vi "1_Search string and replace.vi"() -> ()   [LabVIEW 2010]
panel:
  out "String Out":string
  in  "New Character":string="sleeping"
  in  "Pattern or Character to Replace":string="lazy"
  in  "String In":string="The quick brown fox jumped over the lazy dog."
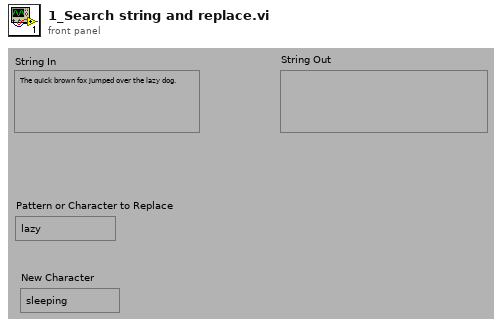
[diagram p1: front panel]
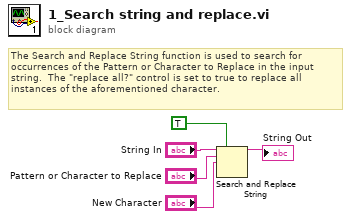
[diagram p0: block diagram]
diagram:
  # "The Search and Replace String function is used to search for \noccurrences of the Pattern or Character to Replace in the input \nstring.  The \"replace all?\" control is set to true to replace all \ninstances of the aforementioned character."
  n1 = Search and Replace String(replace all?=TRUE ("replace all? (F)"), input string="String In", search string="Pattern or Character to Replace", replace string="New Character") -> (result string=→"String Out":string)  [unwired: 4 in, 3 out]
